vi "Read String from String Array.vi"(2 "error in (no error)":errorcluster, 3 "Variables":string[](array[string]), 4 "Name":string) -> (0 "error out":errorcluster, 1 "Variable":string)   [LabVIEW 2014]
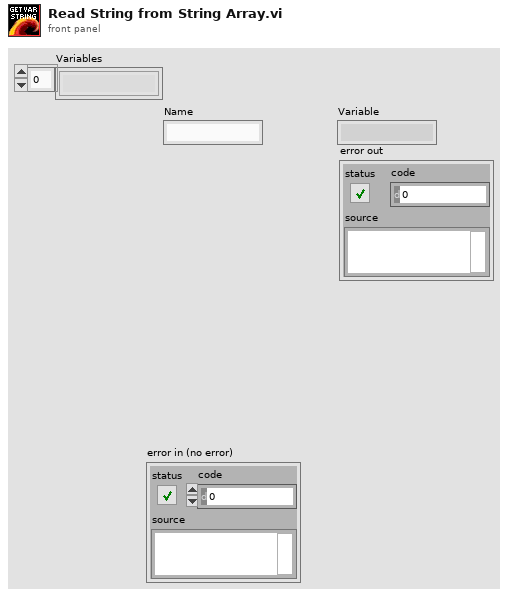
[diagram p1: front panel]
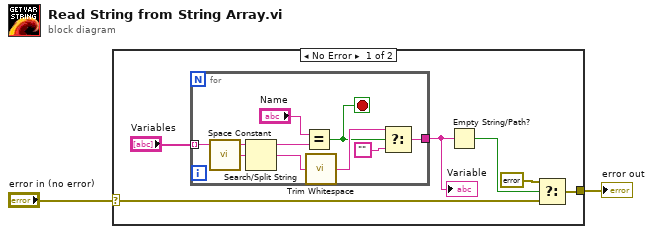
[diagram p0: block diagram]
diagram:
  n1 = case shown="No Error" "error in (no error)" {
    selector: "error in (no error)" -> [w5 w18]
    tunnel: [w4 w18] -> w1
    frame No Error {
      n2 = for {
        tunnel: [w10] -> w8
        tunnel: "Variables" -> [w9] mode=indexing
        stop <- w11 stop-if-true
        n3 = call <vilib>:"Space Constant.vi"() -> ("String"=w17:string)
        n4 = Search/Split String(string=w9, search string/char (-)=w17) -> (substring before match=w15:string, match + rest of string=w16:string)  [unwired: 1 in, 1 out]
        n5 = Equal?(x="Name", y=w15) -> (x = y?=w11:bool)
        n6 = call <vilib>:"Trim Whitespace.vi"("string"=w16) -> ("trimmed string"=w13:string)  [unwired: 1 in]
        n7 = Select(t=w13, s=w11, f="") -> (s? t:f=w10:string)
      }
      "Variable" <- w8
      n8 = Empty String/Path?(string/path=w8) -> (empty?=w7:bool)
      n9 = Select(t=errorcluster {"status"=TRUE, "code"=0, "source"="Variable\nnot found"} ("error constant"), s=w7, f=w5) -> (s? t:f=w4:errorcluster)
    }
    frame Error {
    }
  }
  "error out" <- w1
